vi "VIPB Build UI.vi"() -> ()   [LabVIEW 2014, in "VIPB Build Node.lvclass"]
uses:
  VIPB Build Node.lvclass
  <vilib>/NI/Configuration Framework/Node/NodeRef.ctl
  <vilib>/ni/Configuration Framework/Node/NISE_CEF_Node.lvclass
  <vilib>/NI/AMC/Message Queue.ctl
  <vilib>/NI/AMC/Message.ctl
  <vilib>/NI/Tools/Keyed Array/KeyedArray.ctl
  <vilib>/NI/Configuration Framework/Node/UserEventRef.ctl
  <vilib>/NI/Configuration Framework/Controls/EventCluster.ctl
  VIPB Build Node.lvclass/VIPB Build Node.ctl
  Classes/Build Job/Build Job.lvclass/Build Job.ctl
  <vilib>/NI/AMC/Create Single Message.vi
  <vilib>/NI/AMC/Update Message Routing Info.vi
  <vilib>/NI/AMC/Send Message.vi
  Classes/Build Job/Build Job.lvclass
  <vilib>/NI/AMC/AMC.lvlib
  <vilib>/NI/Tools/Keyed Array/Tools_KeyedArray.lvlib
  <vilib>/NI/Configuration Framework/NISE_CEF_TreeControl.lvlib
panel:
  in  "LabVIEW Version (14.0 format)":string="14.0"
  in  "Install after build?":bool
  in  "user event":T1
  in  "main queue":T2
  in  "VIPB Path":path=path "C:/Projects/LabVIEW Continuous Integration/LabVIEW Continuous Integration.lvproj"
  in  "Description":string
  in  "node ref":T3
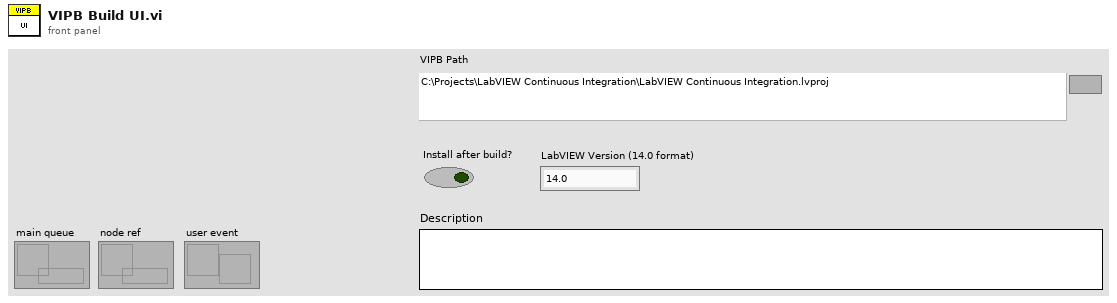
[diagram p1: front panel]
types:
  T1 = typedef "NISE_CEF_Node.lvclass/UserEventRef.ctl" = refnum<user-event>
  T2 = typedef "AMC.lvlib/Message Queue.ctl" = refnum<queue>
  T3 = typedef "NISE_CEF_Node.lvclass/NodeRef.ctl" = refnum<data-value>
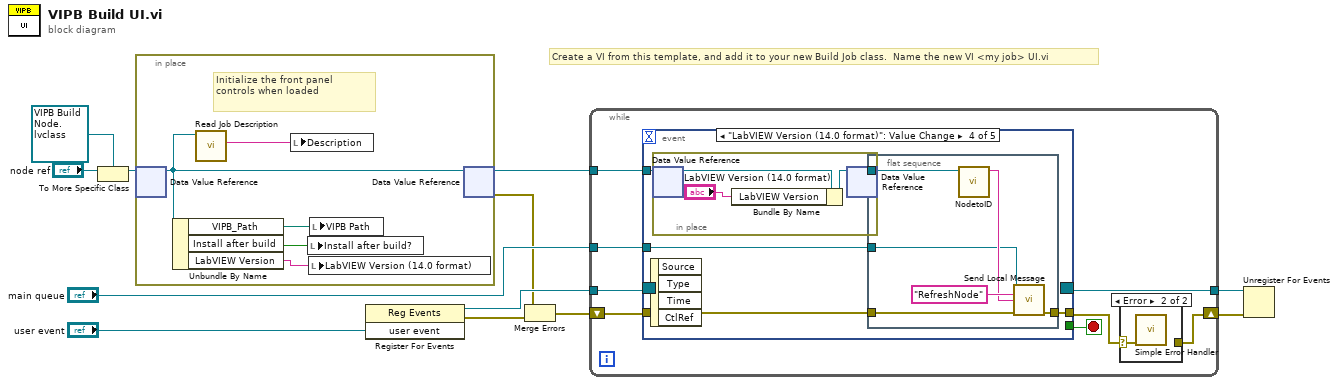
[diagram p0: block diagram]
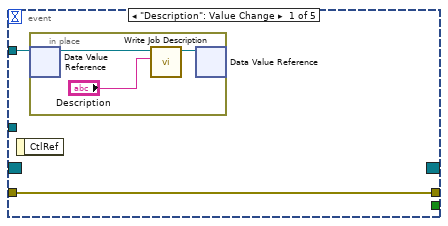
[diagram p3: hidden frame]
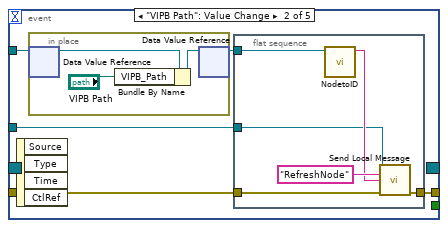
[diagram p4: hidden frame]
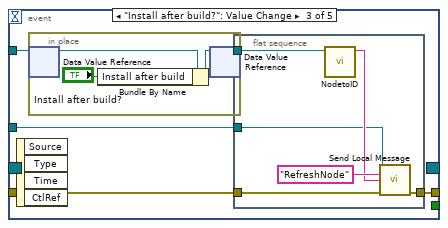
[diagram p5: hidden frame]
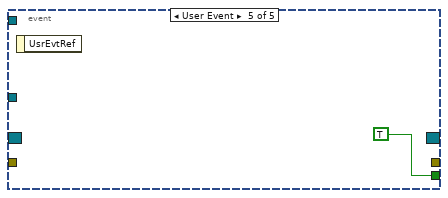
[diagram p6: hidden frame]
diagram:
  # "Create a VI from this template, and add it to your new Build Job class.  Name the new VI <my job> UI.vi"
  n1 = To More Specific Class(target class=refnum<data-value> refnum ("data value reference"), reference="node ref") -> (specific class reference=w6:refnum<data-value>)  [unwired: 1 in, 1 out]
  n2 = in-place {
    # "Initialize the front panel controls when loaded"
    n3 = in-place-dvr #1(w6) -> (w16:refnum<class "VIPB Build Node.lvclass">)  [unwired: 1 out]
    n4 = Unbundle By Name(w16) -> ("VIPB_Path"=w15:path, "Install after build"=w14:bool, "LabVIEW Version"=w13:string)
    n5 = call-dynamic "Read Job Description.vi"("Build Job in"=w16) -> ("Job Description"=w17:string)  [unwired: 10 in]
    n6 = local write "Description"(w17) -> ()
    n7 = local write "Install after build?"(w14) -> ()
    n8 = local write "LabVIEW Version (14.0 format)"(w13) -> ()
    n9 = local write "VIPB Path"(w15) -> ()
    n10 = in-place-dvr #1(w16) -> (w2:refnum<data-value>, w4:errorcluster)
  }
  n11 = register-events("user event") -> (reference out=w10:refnum<event-registration>, error out=w5:errorcluster)  [unwired: 2 in]
  n12 = Merge Errors(w4, w5) -> (w3:errorcluster)
  n13 = while {
    tunnel: w2 -> [w25]
    tunnel: "main queue" -> [w24]
    tunnel: w10 -> [w23]
    tunnel: [w22] -> w9
    shift-right: [w18] -> w8
    shift-left: w3 -> [w21]
    stop <- w20 stop-if-true
    n14 = event shown="[3] \"LabVIEW Version (14.0 format)\": Value Change" {
      selector: w23 -> [_ _ _ _ _]
      dyn-events: [_ _ _ _ _] -> w22
      timeout: _ -> [_ _ _ _ _]
      tunnel: w25 -> [w29 w37 w51 w65 _]
      tunnel: w24 -> [_ w33 w47 w61 _]
      tunnel: [_ _ _ _ TRUE] -> w20
      tunnel: [w28 w34 w48 w62 _] -> w19
      tunnel: w21 -> [w28 w35 w49 w63 _]
      event "Description": Value Change {
        n15 = event-data() -> ()  [unwired: 1 in, 1 out]
        n16 = in-place {
          n17 = in-place-dvr #2(w29) -> (w32:refnum<class "VIPB Build Node.lvclass">)  [unwired: 1 out]
          n18 = call "Write Job Description.vi"("Job Description"="Description", "Build Job in"=w32) -> ("Build Job out"=w31:refnum<class "VIPB Build Node.lvclass">)  [unwired: 9 in]
          n19 = in-place-dvr #2(w31) -> ()  [unwired: 2 out]
        }
      }
      event "VIPB Path": Value Change {
        n20 = event-data() -> ()  [unwired: 1 in, 4 out]
        n21 = in-place {
          n22 = in-place-dvr #3(w37) -> (w46:refnum<class "VIPB Build Node.lvclass">)  [unwired: 1 out]
          n23 = Bundle By Name(cluster=w46, "VIPB_Path"="VIPB Path") -> (w45:refnum<class "VIPB Build Node.lvclass">)
          n24 = in-place-dvr #3(w45) -> (w36:refnum<data-value>)  [unwired: 1 out]
        }
        n25 = flat-sequence {
          tunnel: w36 -> [w41]
          tunnel: w35 -> [w40]
          tunnel: [w39] -> w34
          tunnel: w33 -> [w38]
          frame #0 {
            n26 = call <vilib>:"NodetoID.vi"("node ref"=w41) -> ("ID"=w42:string)  [unwired: 9 in, 1 out]
            n27 = call <vilib>:"Send Local Message.vi"("message queue in"=w38, "message name"="RefreshNode" ("Message Name"), "message value"=w42, "error in"=w40) -> ("error out"=w39:errorcluster)  [unwired: 9 in, 2 out]
          }
        }
      }
      event "Install after build?": Value Change {
        n28 = event-data() -> ()  [unwired: 1 in, 4 out]
        n29 = in-place {
          n30 = in-place-dvr #4(w51) -> (w60:refnum<class "VIPB Build Node.lvclass">)  [unwired: 1 out]
          n31 = Bundle By Name(cluster=w60, "Install after build"="Install after build?") -> (w59:refnum<class "VIPB Build Node.lvclass">)
          n32 = in-place-dvr #4(w59) -> (w50:refnum<data-value>)  [unwired: 1 out]
        }
        n33 = flat-sequence {
          tunnel: w50 -> [w55]
          tunnel: w49 -> [w54]
          tunnel: [w53] -> w48
          tunnel: w47 -> [w52]
          frame #0 {
            n34 = call <vilib>:"NodetoID.vi"("node ref"=w55) -> ("ID"=w56:string)  [unwired: 9 in, 1 out]
            n35 = call <vilib>:"Send Local Message.vi"("message queue in"=w52, "message name"="RefreshNode" ("Message Name"), "message value"=w56, "error in"=w54) -> ("error out"=w53:errorcluster)  [unwired: 9 in, 2 out]
          }
        }
      }
      event "LabVIEW Version (14.0 format)": Value Change {
        n36 = event-data() -> ()  [unwired: 1 in, 4 out]
        n37 = in-place {
          n38 = in-place-dvr #5(w65) -> (w74:refnum<class "VIPB Build Node.lvclass">)  [unwired: 1 out]
          n39 = Bundle By Name(cluster=w74, "LabVIEW Version"="LabVIEW Version (14.0 format)") -> (w73:refnum<class "VIPB Build Node.lvclass">)
          n40 = in-place-dvr #5(w73) -> (w64:refnum<data-value>)  [unwired: 1 out]
        }
        n41 = flat-sequence {
          tunnel: w64 -> [w69]
          tunnel: w63 -> [w68]
          tunnel: [w67] -> w62
          tunnel: w61 -> [w66]
          frame #0 {
            n42 = call <vilib>:"NodetoID.vi"("node ref"=w69) -> ("ID"=w70:string)  [unwired: 9 in, 1 out]
            n43 = call <vilib>:"Send Local Message.vi"("message queue in"=w66, "message name"="RefreshNode" ("Message Name"), "message value"=w70, "error in"=w68) -> ("error out"=w67:errorcluster)  [unwired: 9 in, 2 out]
          }
        }
      }
      event User Event {
        n44 = event-data() -> ()  [unwired: 1 in, 1 out]
      }
    }
    n45 = case shown="Error" w19 {
      selector: w19 -> [w26 w27]
      tunnel: [w26 _] -> w18
      frame No Error {
      }
      frame Error {
        n46 = call <vilib>:"Simple Error Handler.vi"("error in (no error)"=w27) -> ()  [unwired: 4 in, 5 out]
      }
    }
  }
  n47 = Unregister For Events(event registration refnum=w9, error in=w8) -> ()  [unwired: 1 out]
